vi "backproject.vi"(9 "Keep pixels?":bool, 10 "Image Properties":T4, 11 "Backproject Input":T1) -> (1 "Projection Pixels":T2(array[cluster]), 2 "Projections":T3[](array[typedef]), 3 "Output":sgl[](array[numeric]))   [LabVIEW 2013]
uses:
  tags_cluster.ctl
  bp_work_unit.ctl
  backproject_input.ctl
  pixels_for_proj.ctl
panel:
  out "Normalisation":i32[](array[numeric])
  out "Current summing work unit #":i32
  out "destroyed queue name":string
  out "Selector":dbl
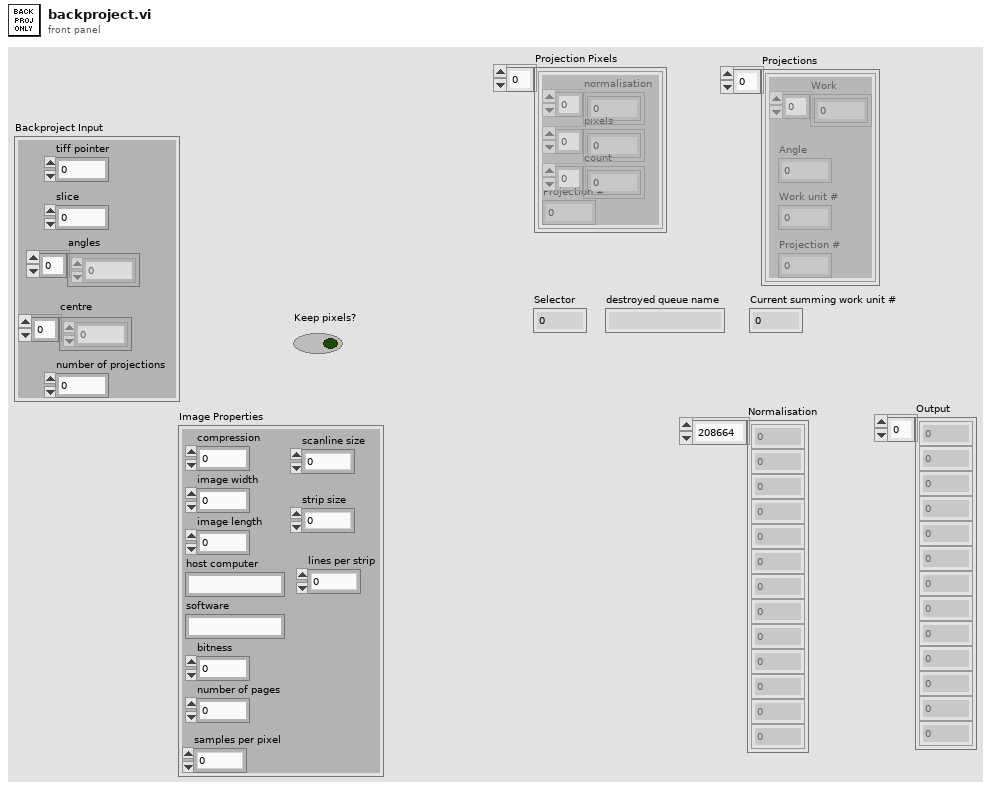
[diagram p1: front panel]
types:
  T1 = typedef "backproject_input.ctl" = cluster{"tiff pointer":i64, "slice":u32, "angles":dbl[], "centre":i32[], "number of projections":u32}
  T2 = cluster{"normalisation":i32[], "pixels":i32[], "count":i32[], "Projection #":i32}[]
  T3 = typedef "bp_work_unit.ctl" = cluster{"Work":u8[], "Angle":dbl, "Work unit #":i32, "Projection #":i32}
  T4 = typedef "tags_cluster.ctl" = cluster{"compression":i32, "image width":i32, "image length":i32, "host computer":string, "software":string, "bitness":i32, "number of pages":i32, "samples per pixel":i32, "scanline size":i32, "strip size":i32, "lines per strip":i32}
  T5 = typedef "pixels_for_proj.ctl" = cluster{"normalisation":i32[], "pixels":i32[], "count":i32[], "Projection #":i32}
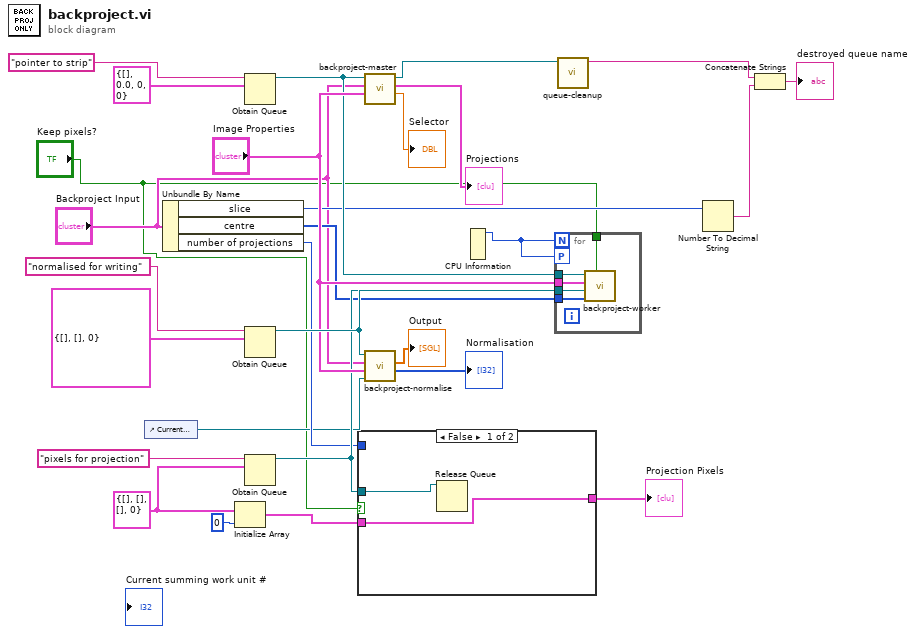
[diagram p0: block diagram]
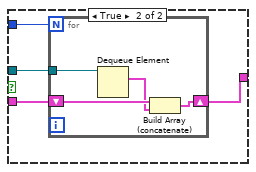
[diagram p2: hidden frame]
diagram:
  w15 = T5 {"normalisation"=[], "pixels"=[], "count"=[], "Projection #"=0}
  n1 = control-ref of="Current summing work unit #"() -> (w3:refnum<vi>)
  n2 = Unbundle By Name("Backproject Input") -> ("slice"=w8:u32, "centre"=w7:i32[], "number of projections"=w5:u32)
  n3 = Initialize Array(w15, 0 ("dimension size")) -> (w13:T5[])
  n4 = Obtain Queue(name (unnamed)="pointer to strip", element data type=T3 {"Work"=[], "Angle"=0.0, "Work unit #"=0, "Projection #"=0} ("backproject work unit")) -> (queue out=w11:refnum<queue>)  [unwired: 3 in, 2 out]
  n5 = Obtain Queue(name (unnamed)="normalised for writing", element data type=cluster{sgl[], i32[], i32} {[], [], 0}) -> (queue out=w24:refnum<queue>)  [unwired: 3 in, 2 out]
  n6 = Obtain Queue(name (unnamed)="pixels for projection", element data type=w15) -> (queue out=w16:refnum<queue>)  [unwired: 3 in, 2 out]
  n7 = case shown="False" "Keep pixels?" {
    tunnel: w16 -> [w30 w34]
    tunnel: w13 -> [w29 w33]
    tunnel: [w29 w32] -> w12
    tunnel: w5 -> [_ w31]
    frame False {
      n8 = Release Queue(queue=w30) -> ()  [unwired: 2 in, 3 out]
    }
    frame True {
      n9 = for {
        N: w31 -> [_]
        tunnel: w34 -> [w38]
        shift-right: [w36] -> w32
        shift-left: w33 -> [w37]
        n10 = Dequeue Element(queue=w38) -> (element=w35:T5)  [unwired: 2 in, 3 out]
        n11 = Build Array (concatenate)(w37, w35) -> (w36:T5[])
      }
    }
  }
  "Projection Pixels" <- w12
  n12 = call "backproject-master.vi"("Image Properties"="Image Properties", "Backproject Input"="Backproject Input", "Queue in"=w11) -> ("Selector"=→"Selector":dbl, "Projections"=→"Projections":T3[], "Queue out"=w10:refnum<queue>)  [unwired: 6 in]
  n13 = call "backproject-normalise.vi"("Ctl Refnum"=w3, "Image Properties"="Image Properties", "Backproject Input"="Backproject Input", "Queue in"=w24) -> ("Normalisation"=→"Normalisation":i32[], "Array"=→"Output":sgl[])  [unwired: 4 in, 2 out]
  n14 = CPU Information() -> (4:w1:i32)  [unwired: 3 out]
  n15 = for {
    N: w1 -> [_]
    tunnel: w24 -> [w44]
    tunnel: "Image Properties" -> [w43]
    tunnel: w16 -> [w42]
    tunnel: w11 -> [w41]
    tunnel: w7 -> [w40]
    tunnel: "Keep pixels?" -> [w39]
    workers-P: w1 -> [_]
    n16 = call "backproject-worker.vi"("pixels for projections"=w42, "Keep pixels?"=w39, "Centre"=w40, "Write queue"=w44, "Image Properties"=w43, "Work queue in"=w41) -> ()  [unwired: 3 in, 3 out]
  }
  n17 = call "queue-cleanup.vi"("Queue in"=w10) -> ("queue name"=w19:string)  [unwired: 10 in]
  n18 = Number To Decimal String(number=w8) -> (decimal integer string=w18:string)  [unwired: 1 in]
  n19 = Concatenate Strings(w19, w18) -> (→"destroyed queue name":string)
